vi "ResetPositionGlobals.vi"(8 "error in":errorcluster) -> (0 "error out":errorcluster)   [LabVIEW 2014]
uses:
  Gantry/GantryGlobals.vi
  Automated Tasks/AutomationGlobals.vi
  Automated Tasks/ToteCount.vi
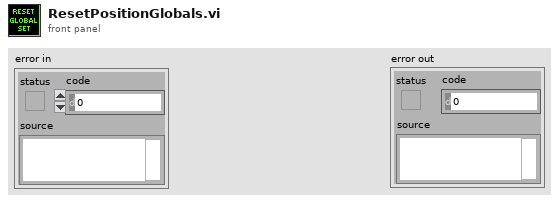
[diagram p1: front panel]
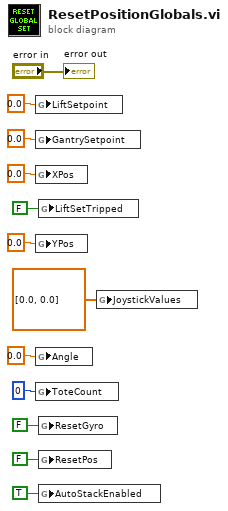
[diagram p0: block diagram]
diagram:
  n1 = global write "GantryGlobals.vi" "LiftSetpoint"(0.0 ("LiftSetpoint")) -> ()
  n2 = global write "GantryGlobals.vi" "GantrySetpoint"(0.0 ("LiftSetpoint")) -> ()
  n3 = global write "AutomationGlobals.vi" "XPos"(0.0 ("XPos")) -> ()
  n4 = global write "AutomationGlobals.vi" "YPos"(0.0 ("XPos")) -> ()
  n5 = global write "AutomationGlobals.vi" "Angle"(0.0 ("XPos")) -> ()
  n6 = global write "ToteCount.vi" "ToteCount"(0 ("ToteCount")) -> ()
  n7 = global write "GantryGlobals.vi" "LiftSetTripped"(FALSE ("LiftSetTripped")) -> ()
  n8 = global write "AutomationGlobals.vi" "ResetGyro"(FALSE ("ResetGyro")) -> ()
  n9 = global write "AutomationGlobals.vi" "ResetPos"(FALSE ("ResetGyro")) -> ()
  n10 = global write "AutomationGlobals.vi" "AutoStackEnabled"(TRUE ("AutoStackEnabled")) -> ()
  n11 = global write "AutomationGlobals.vi" "JoystickValues"(dbl[] [0.0, 0.0] ("s? t:f")) -> ()
  "error out" <- "error in"
